vi "lisa_functional_2.vi"() -> ()   [LabVIEW 2019]
doc: "The classic \"Hello World\" example."
uses:
  <vilib>/Enthought/Python Integration Toolkit/Python Integration Toolkit.lvlib
  <vilib>/Enthought/Python Integration Toolkit/api/Unpack String.vi
  <vilib>/Analysis/Matrix/Datatypes/ComplexMatrix.ctl
  <vilib>/Analysis/Matrix/NI_Matrix.lvlib
panel:
  in  "b (t)":dbl
  in  "a (t)":dbl
  in  "D y":dbl
  in  "D x":dbl
  in  "Static Offsets":dbl
  in  "Arm Length [m]":dbl
  in  "Magnification":dbl
  in  "D y":dbl
  in  "Argument":variant
  out "Value":string
  in  "d x 2":dbl
  in  "Scatter. matrix 2":T1
  in  "Mode Coeff. (Cnm) 2":T1
  in  "Beam Param. 2":cdb
  in  "D x":dbl
  in  "Arm Length":dbl
  in  "Scatter. matrix":T1
  in  "Mode Coeff. (Cnm)":T1
  in  "Beam Param.":cdb
  # "Dynamic offsets"
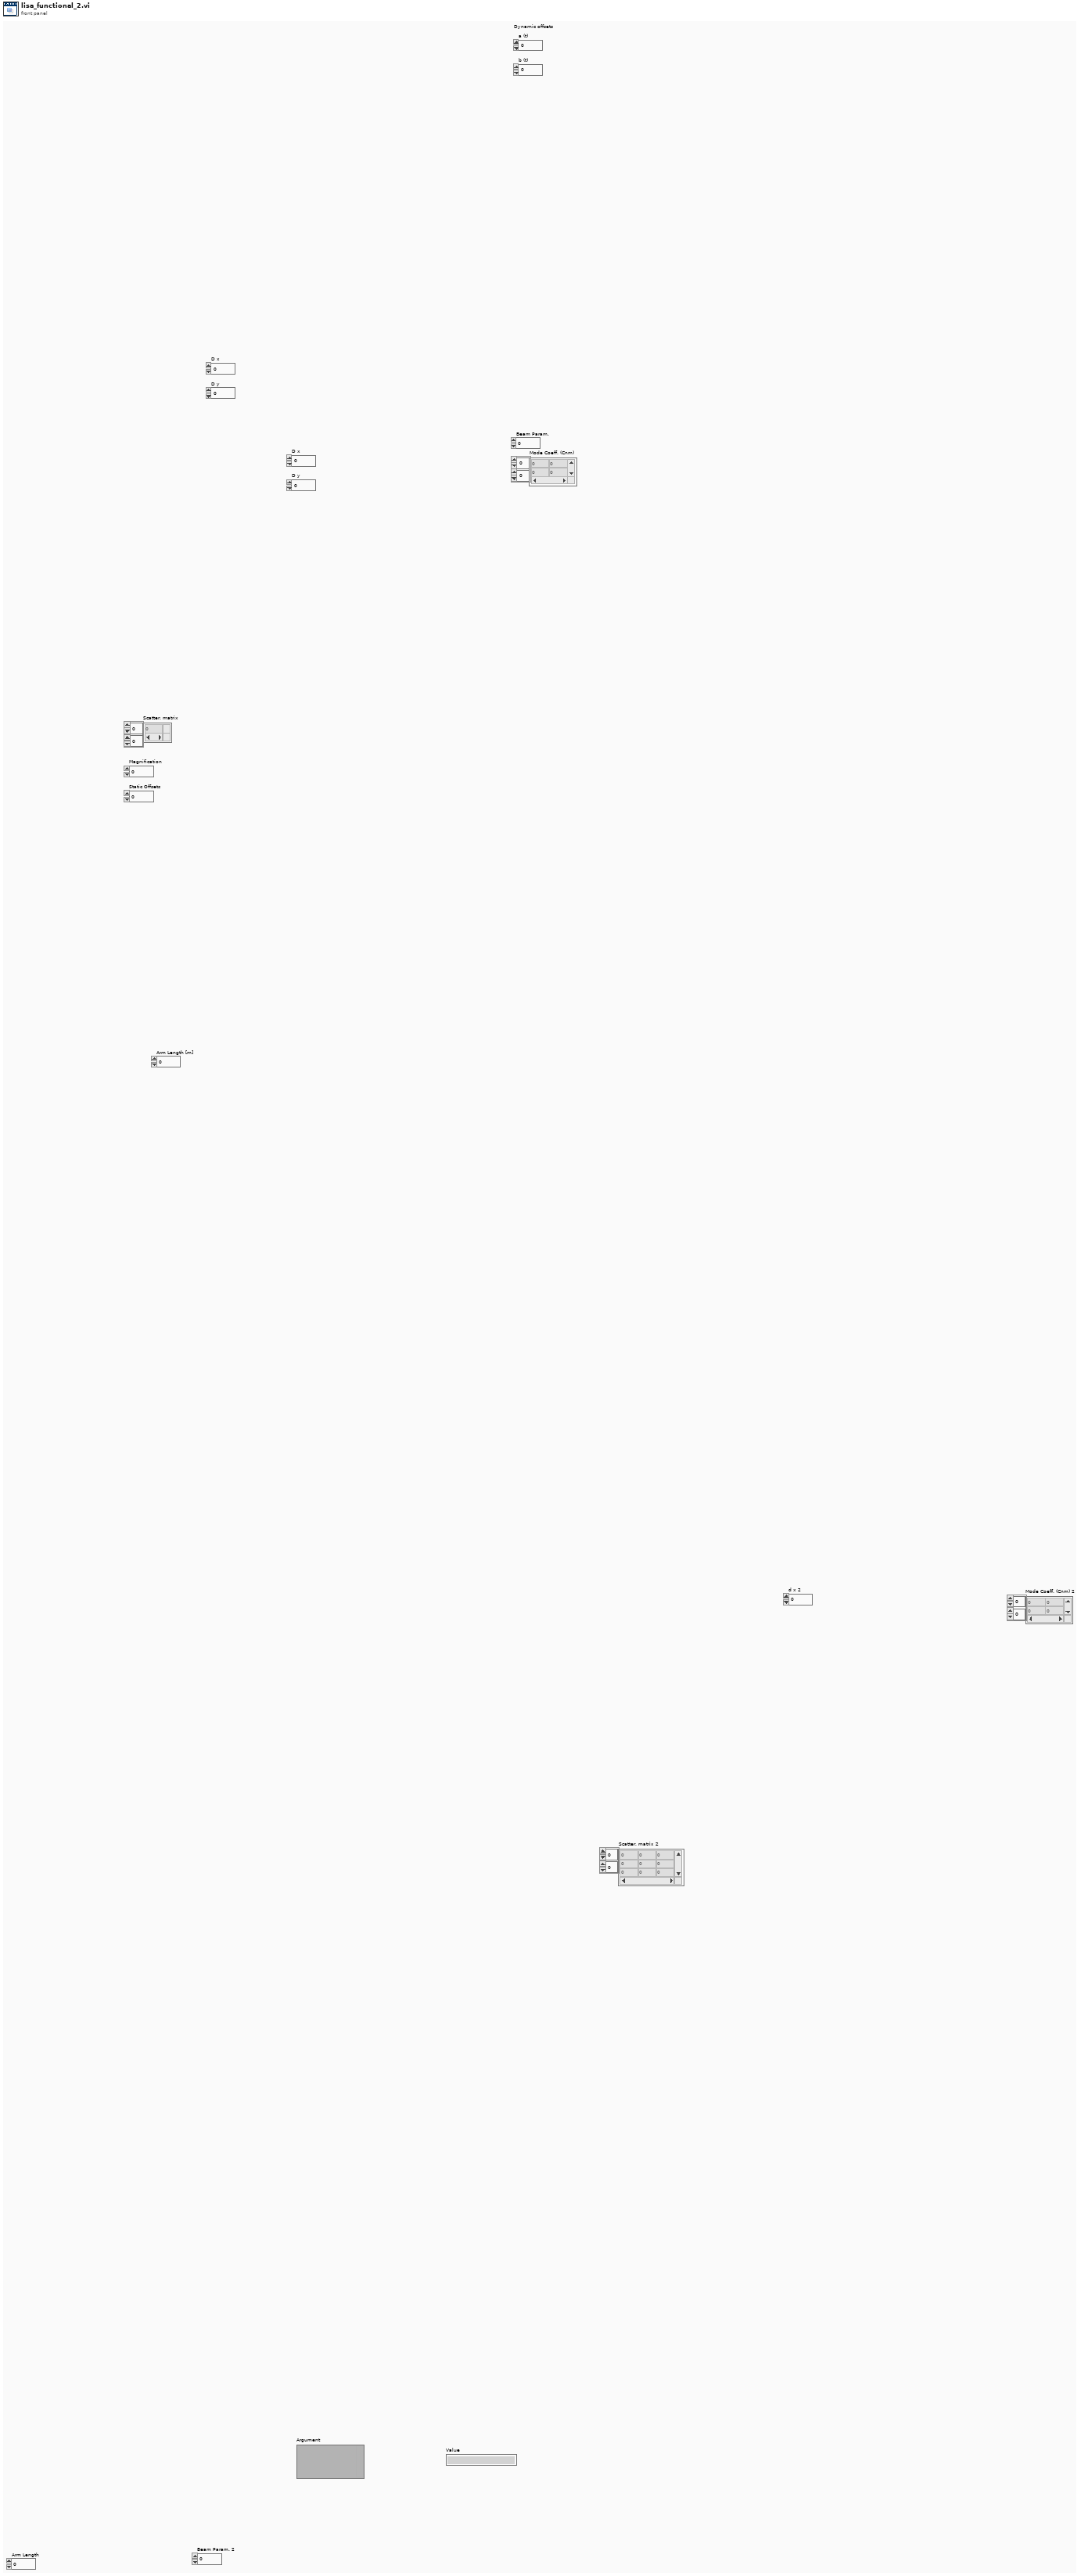
[diagram p1: front panel]
types:
  T1 = typedef "NI_Matrix.lvlib/ComplexMatrix.ctl" = cdb[][]
  T2 = typedef "Python Integration Toolkit.lvlib/Session ID.ctl" = u64
  T3 = typedef "Python Integration Toolkit.lvlib/Console Visibility.ctl" = enum16{"Show Console", "Show Console While Running", "Hide Console"}
  T4 = typedef "Python Integration Toolkit.lvlib/Python Objects.ctl" = variant
  T5 = cluster{"Beam Param.":cdb, "Mode Coeff. (Cnm)":T1}
  T6 = cluster{cluster{"Beam Param.":cdb, "Mode Coeff. (Cnm)":T1}, "D x":dbl}
  T7 = cluster{cluster{cluster{"Beam Param.":cdb, "Mode Coeff. (Cnm)":T1}, "D x":dbl}, "Scatter. matrix":T1}
diagram:
  # "LASER"
  # "TS"
  # "OB"
  # "TS 1"
  # "S/C 2"
  # "OB 1"
  # "S/C 1"
  # "Laser 1"
  # "Finally, we close the connection.  This\nwill exit Python."
  # "Turn the Python function result\ninto LabVIEW data."
  # "Call the Python function and\ncollect the result."
  # "We're going to make a Python function call, which takes one\nargument: the user's name.  This prepares the data to be sent\nto Python."
  # "Then we load the module and start Python.  This\nreturns a Session ID, which we supply to the other\nsubVI's to perform tasks."
  # "First we need the absolute path to the Python module.\nIn this example, it's in the same folder as the VI."
  n1 = Current VI's Path() -> (path=w29:path)
  n2 = Strip Path(path=w29) -> (stripped path=w28:path)  [unwired: 1 out]
  n3 = Build Path(base path=w28, name or relative path="hello.py") -> (appended path=w26:path)
  n4 = call <vilib>:"New Session.vi"("Path to Python Module (.py File)"=w26) -> ("error out"=w18:errorcluster, "Session ID out"=w19:T2, "Console Visibility"=w13:T3)  [unwired: 8 in]
  n5 = call <vilib>:"Pack.vi"("Argument"="Argument", "error in (no error)"=w18, "Session ID"=w19) -> ("error out"=w16:errorcluster, "Python Object References Out"=w14:T4, "Session ID out"=w17:T2)  [unwired: 6 in]
  n6 = call <vilib>:"Call.vi"("Function or Method Name"="say_hello", "error in (no error)"=w16, "Python Object References In"=w14, "Session ID"=w17) -> ("error out"=w24:errorcluster, "Python Object References Out"=w21:T4, "Session ID out"=w25:T2)  [unwired: 5 in]
  n7 = call-poly <vilib>:"Unpack.vi"("error in (no error)"=w24, "Python Object References In"=w21, "Session ID"=w25) -> ("error out"=w22:errorcluster, "Value"=→"Value":string, "Session ID out"=w23:T2)  [unwired: 5 in, 1 out]
  n8 = Bundle "function foo"("Beam Param."="Beam Param.", "Mode Coeff. (Cnm)"="Mode Coeff. (Cnm)") -> (w12:T5)  [unwired: 1 in]
  n9 = call <vilib>:"Close Session.vi"("error in (no error)"=w22, "Session ID"=w23) -> ()  [unwired: 9 in, 1 out]
  n10 = Bundle "function bar"(w12, "D x"="D x") -> (w8:T6)  [unwired: 1 in]
  n11 = Bundle "function bar"("d x 2"="d x 2", "d x 2"="d x 2") -> ()  [unwired: 1 in, 1 out]
  n12 = Bundle "function foo"(w8, "Scatter. matrix"="Scatter. matrix") -> (w6:T7)  [unwired: 1 in]
  n13 = Bundle "function foo"(w6, "Arm Length"="Arm Length") -> ()  [unwired: 1 in, 1 out]
  n14 = Bundle "function foo"("d x 2", "Beam Param. 2"="Beam Param. 2", "Mode Coeff. (Cnm) 2"="Mode Coeff. (Cnm) 2") -> ()  [unwired: 1 in]
  n15 = call "lisa_functional_2.vi"() -> ()  [unwired: 12 in]
